vi "Install LVClassLibrary Tools.vi"(11 "Files Installed":path[](array[path])) -> ()   [LabVIEW 2020]
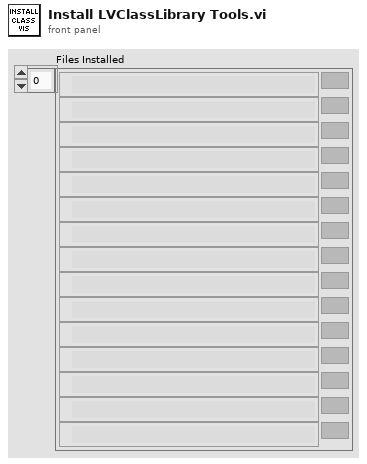
[diagram p1: front panel]
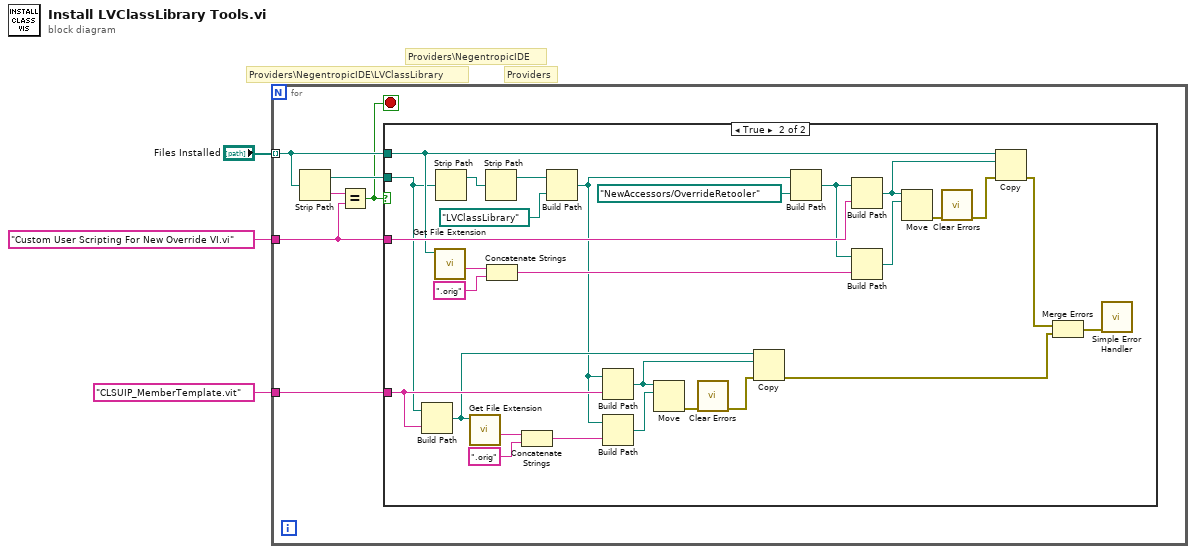
[diagram p0: block diagram]
diagram:
  # "Providers"
  # "Providers\\NegentropicIDE"
  # "Providers\\NegentropicIDE\\LVClassLibrary"
  n1 = for {
    tunnel: "Files Installed" -> [w9] mode=indexing
    tunnel: "Custom User Scripting For New Override VI.vi" -> [w4]
    tunnel: "CLSUIP_MemberTemplate.vit" -> [w5]
    stop <- w7 stop-if-true
    n2 = Strip Path(path=w9) -> (stripped path=w8:path, name=w6:string)
    n3 = Equal?(x=w6, y=w4) -> (x = y?=w7:bool)
    n4 = case shown="True" w7 {
      tunnel: w9 -> [_ w33]
      tunnel: w8 -> [_ w16]
      tunnel: w4 -> [_ w34]
      tunnel: w5 -> [_ w23]
      frame False {
      }
      frame True {
        n5 = Build Path(base path=w16, name or relative path=w23) -> (appended path=w21:path)
        n6 = call <vilib>:"Get File Extension.vi"("file"=w33) -> ("filename without extension"=w32:string)  [unwired: 6 in, 4 out]
        n7 = Strip Path(path=w16) -> (stripped path=w37:path)  [unwired: 1 out]
        n8 = call <vilib>:"Get File Extension.vi"("file"=w21) -> ("filename without extension"=w25:string)  [unwired: 6 in, 4 out]
        n9 = Strip Path(path=w37) -> (stripped path=w36:path)  [unwired: 1 out]
        n10 = Concatenate Strings(w32, ".orig" ("string")) -> (w30:string)
        n11 = Concatenate Strings(w25, ".orig" ("string")) -> (w24:string)
        n12 = Build Path(base path=w36, name or relative path=path "LVClassLibrary") -> (appended path=w18:path)
        n13 = Build Path(base path=w18, name or relative path=w23) -> (appended path=w20:path)
        n14 = Build Path(base path=w18, name or relative path=w24) -> (appended path=w22:path)
        n15 = Move(source path=w20, 10:w22) -> (error out=w19:errorcluster)  [unwired: 3 in, 2 out]
        n16 = call <vilib>:"Clear Errors.vi"("error in (no error)"=w19) -> ("error out"=w14:errorcluster)  [unwired: 5 in, 1 out]
        n17 = Copy(8:w14, 10:w20, 11:w21) -> (0:w11:errorcluster)  [unwired: 2 in, 2 out]
        n18 = Build Path(base path=w18, name or relative path=path "NewAccessors/OverrideRetooler") -> (appended path=w15:path)
        n19 = Build Path(base path=w15, name or relative path=w34) -> (appended path=w28:path)
        n20 = Build Path(base path=w15, name or relative path=w30) -> (appended path=w29:path)
        n21 = Move(source path=w28, 10:w29) -> (error out=w27:errorcluster)  [unwired: 3 in, 2 out]
        n22 = call <vilib>:"Clear Errors.vi"("error in (no error)"=w27) -> ("error out"=w13:errorcluster)  [unwired: 5 in, 1 out]
        n23 = Copy(8:w13, 10:w28, 11:w33) -> (0:w12:errorcluster)  [unwired: 2 in, 2 out]
        n24 = Merge Errors(w12, w11) -> (w10:errorcluster)
        n25 = call <vilib>:"Simple Error Handler.vi"("error in (no error)"=w10) -> ()  [unwired: 4 in, 5 out]
      }
    }
  }
